vi "checknextstep.vi"(10 "Step":i32, 11 "StepNumber":i32[](array[numeric])) -> (2 "Index":i32, 3 "ok":bool)   [LabVIEW 2019, in "MPC_VirbVision.lvclass"]
uses:
  MPC_VirbVision.lvclass
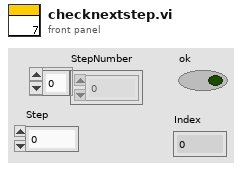
[diagram p1: front panel]
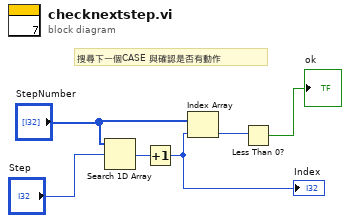
[diagram p0: block diagram]
diagram:
  # "搜尋下一個CASE 與確認是否有動作"
  n1 = Search 1D Array(1D array="StepNumber", element="Step") -> (index of element=w2:i32)  [unwired: 1 in]
  n2 = Increment(x=w2) -> (x+1=w5:i32)
  "Index" <- w5
  n3 = Index Array(array="StepNumber", index=w5) -> (element=w3:i32)
  n4 = Less Than 0?(x=w3) -> (x < 0?=→"ok":bool)
